vi "file_configuration.vi"(4 "force_read?":bool, 6 "custom_file":path, 7 "command":T1=enum."read_config", 8 "error in (no error)":errorcluster, 10 "project_file":path, 11 "config in":T2) -> (0 "error out":errorcluster, 3 "config out":T2)   [LabVIEW 2015, in "lv-builder-default.lvlib"]
doc: "This VI is able to read/write configuration from all the associated modules defined in the master data cluster. It also acts as a functional global/data store in the event that no data has changed since the last write. It will self-initialize and well set an internal flag in the event an error is encountered when reading. If no command is provided, it will default to the read command."
uses:
  lv-builder-default.lvlib
  _controls/configuration.ctl
  _controls/command_configuration.ctl
  lv-build/lv-build.lvlib
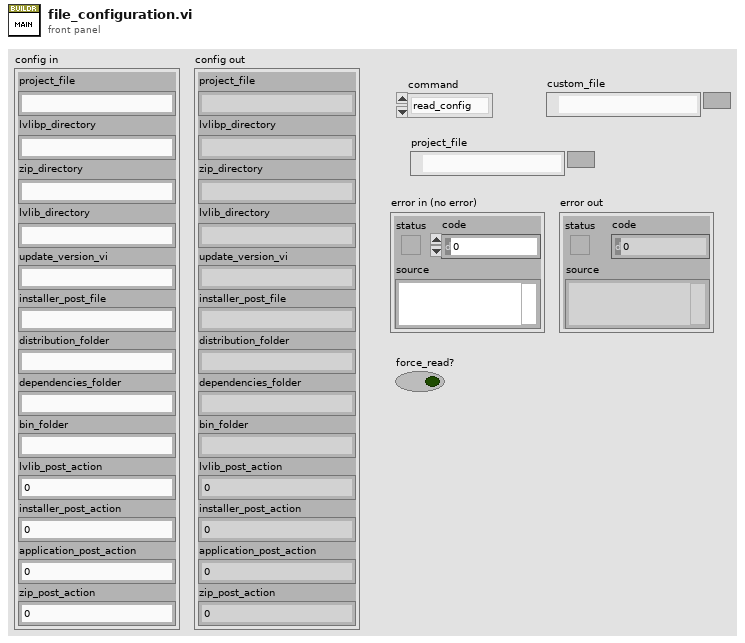
[diagram p1: front panel]
types:
  T1 = typedef "lv-builder-default.lvlib/command_configuration.ctl" = enum16{"<config_command>", "read_config", "write_config", "<null>"}
  T2 = typedef "lv-builder-default.lvlib/configuration.ctl" = cluster{"project_file":string, "lvlibp_directory":string, "zip_directory":string, "lvlib_directory":string, "update_version_vi":string, "installer_post_file":string, "distribution_folder":string, "dependencies_folder":string, "bin_folder":string, "lvlib_post_action":u16, "installer_post_action":u16, "application_post_action":u16, "zip_post_action":u16}
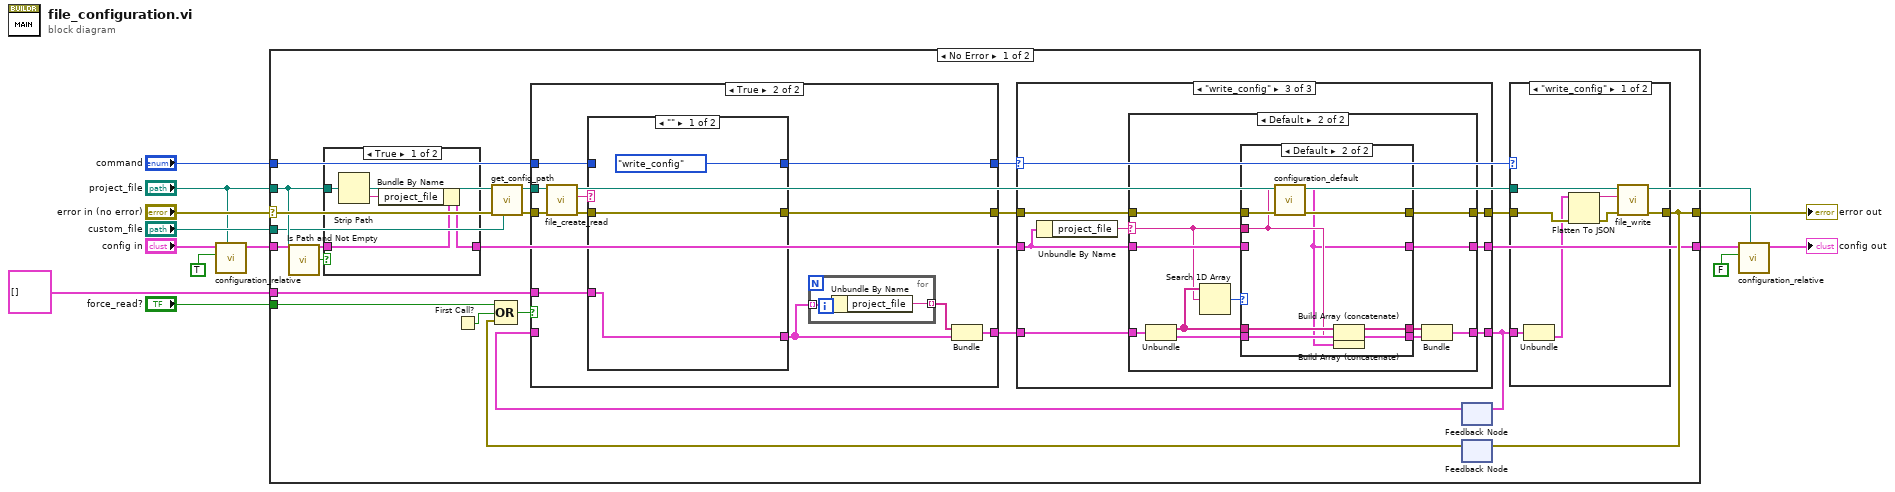
[diagram p0: block diagram]
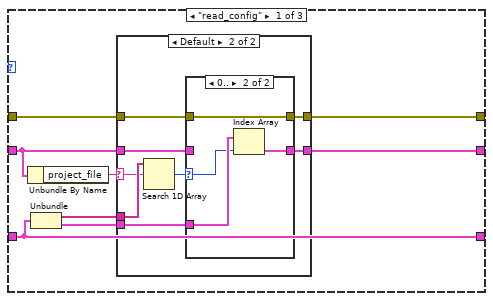
[diagram p3: hidden frame]
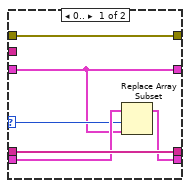
[diagram p8: hidden frame]
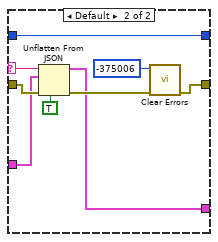
[diagram p10: hidden frame]
diagram:
  n1 = call "configuration_relative.vi"("project_file"="project_file", "to_relative"=TRUE, "configuration in"="config in") -> ("configuration out"=w3:T2)  [unwired: 8 in]
  n2 = case shown="No Error" "error in (no error)" {
    selector: "error in (no error)" -> [w19 w139]
    tunnel: "command" -> [w28 _]
    tunnel: [w35 w139] -> w10
    tunnel: w3 -> [w21 _]
    tunnel: "custom_file" -> [w14 _]
    tunnel: [w26 _] -> w6
    tunnel: "force_read?" -> [w32 _]
    tunnel: T2[] [] ("default") -> [w29 _]
    tunnel: "project_file" -> [w15 _]
    frame No Error {
      n3 = call <vilib>:"Is Path and Not Empty.vi"("path"=w15) -> ("Is Path and Not Empty?"=w16:bool)  [unwired: 4 in]
      n4 = case shown="True" w16 {
        tunnel: w21 -> [w39 w40]
        tunnel: [w38 w40] -> w17
        tunnel: w15 -> [w37 _]
        frame True {
          n5 = Strip Path(path=w37) -> (name=w36:string)  [unwired: 1 out]
          n6 = Bundle By Name(cluster=w39, "project_file"=w36) -> (w38:T2)
        }
        frame False {
        }
      }
      n7 = First Call?() -> (First Call?: T/F=w33:bool)
      n8 = call "get_config_path.vi"("custom_path"=w14, "error in (no error)"=w19, "project_file"=w15) -> ("error out"=w18:errorcluster, "lv_build_config_path"=w20:path)  [unwired: 7 in]
      n9 = feedback #1() -> (w30:cluster{string[], "default":T2[]})  [unwired: 1 in]
      n10 = feedback #2() -> (w34:errorcluster)  [unwired: 1 in]
      n11 = Compound Arithmetic op=OR(w32, w33, w34) -> (w31:bool)
      n12 = case shown="True" w31 {
        tunnel: w30 -> [w105 _]
        tunnel: w18 -> [w104 w114]
        tunnel: w20 -> [_ w115]
        tunnel: [w104 w112] -> w24
        tunnel: w29 -> [_ w116]
        tunnel: w28 -> [w103 w111]
        tunnel: [w103 w110] -> w25
        tunnel: [w105 w108] -> w27
        frame False {
        }
        frame True {
          n13 = call "file_create_read.vi"("error in (no error)"=w114, "config_path"=w115) -> ("error out"=w113:errorcluster, "string"=w109:string)  [unwired: 8 in]
          n14 = case shown="\"\"" w109 {
            selector: w109 -> [_ w126]
            tunnel: w116 -> [w120 w128]
            tunnel: [w120 w127] -> w107
            tunnel: w113 -> [w121 w130]
            tunnel: [w121 w122] -> w112
            tunnel: w111 -> [_ w125]
            tunnel: [command_configuration."write_config" ("command") w125] -> w110
            frame "" {
            }
            frame Default {
              n15 = Unflatten From JSON(JSON string=w126, type and defaults=w128, default null elements? (F)=TRUE, error in (no error)=w130) -> (value=w127:T2[], error out=w129:errorcluster)  [unwired: 3 in]
              n16 = call <vilib>:"Clear Errors.vi"("error in (no error)"=w129, "specific error code to clear (0: all)"=-375006) -> ("error out"=w122:errorcluster)  [unwired: 4 in, 1 out]
            }
          }
          n17 = for {
            tunnel: w107 -> [w118] mode=indexing
            tunnel: [w117] -> w106 mode=indexing
            n18 = Unbundle By Name(w118) -> ("project_file"=w117:string)
          }
          n19 = Bundle(w106, "default"=w107) -> (w108:cluster{string[], "default":T2[]})  [unwired: 1 in]
        }
      }
      n20 = case shown="\"write_config\"" w25 {
        tunnel: w17 -> [w41 w66 w70]
        tunnel: [w48 w65 w73] -> w22
        tunnel: w27 -> [w48 w65 w71]
        tunnel: [w44 w66 w67] -> w26
        tunnel: w24 -> [w43 w64 w69]
        tunnel: [w42 w64 w68] -> w23
        frame "read_config" {
          n21 = Unbundle By Name(w41) -> ("project_file"=w45:string)
          n22 = Unbundle(w48) -> (w47:string[], "default"=w46:T2[])
          n23 = case shown="Default" w45 {
            selector: w45 -> [_ w54]
            tunnel: w47 -> [_ w57]
            tunnel: w46 -> [_ w56]
            tunnel: [_ w53] -> w44
            tunnel: w43 -> [w49 w52]
            tunnel: [w49 w51] -> w42
            tunnel: w41 -> [_ w50]
            frame "" {
            }
            frame Default {
              n24 = Search 1D Array(1D array=w57, element=w54) -> (index of element=w55:i32)  [unwired: 1 in]
              n25 = case shown="0.." w55 {
                selector: w55 -> [_ w62]
                tunnel: w56 -> [_ w63]
                tunnel: [w58 w61] -> w53
                tunnel: w52 -> [w59 w60]
                tunnel: [w59 w60] -> w51
                tunnel: w50 -> [w58 _]
                frame Default {
                }
                frame 0.. {
                  n26 = Index Array(array=w63, index=w62) -> (element=w61:T2)
                }
              }
            }
          }
        }
        frame Default {
        }
        frame "write_config" {
          n27 = Unbundle By Name(w70) -> ("project_file"=w72:string)
          n28 = case shown="Default" w72 {
            selector: w72 -> [_ w80]
            tunnel: [w76 w86] -> w73
            tunnel: w70 -> [w74 w84]
            tunnel: w71 -> [w76 w82]
            tunnel: w69 -> [w75 w79]
            tunnel: [w75 w78] -> w68
            tunnel: [w74 w77] -> w67
            frame "" {
            }
            frame Default {
              n29 = Unbundle(w82) -> (w81:string[], "default"=w83:T2[])
              n30 = Search 1D Array(1D array=w81, element=w80) -> (index of element=w88:i32)  [unwired: 1 in]
              n31 = case shown="Default" w88 {
                selector: w88 -> [w91 _]
                tunnel: w83 -> [w93 w101]
                tunnel: [w92 w100] -> w87
                tunnel: w81 -> [w94 w98]
                tunnel: [w94 w99] -> w85
                tunnel: w84 -> [w89 _]
                tunnel: w80 -> [_ w96]
                tunnel: w79 -> [w90 w97]
                tunnel: [w90 w102] -> w78
                tunnel: [w89 w95] -> w77
                frame 0.. {
                  n32 = Replace Array Subset(array=w93, new element=w89, index=w91) -> (w92:T2[])
                }
                frame Default {
                  n33 = call "configuration_default.vi"("error in (no error)"=w97, "project_file"=w96) -> ("error out"=w102:errorcluster, "configuration"=w95:T2)  [unwired: 8 in]
                  n34 = Build Array (concatenate)(w98, w96) -> (w99:string[])
                  n35 = Build Array (concatenate)(w101, w95) -> (w100:T2[])
                }
              }
              n36 = Bundle(w85, "default"=w87) -> (w86:cluster{string[], "default":T2[]})  [unwired: 1 in]
            }
          }
        }
      }
      n37 = feedback-in #1(w22) -> ()
      n38 = case shown="\"write_config\"" w25 {
        tunnel: w22 -> [w134 _]
        tunnel: w23 -> [w135 w138]
        tunnel: [w132 w138] -> w35
        tunnel: w20 -> [w133 _]
        frame "write_config" {
          n39 = Unbundle(w134) -> ("default"=w131:T2[])  [unwired: 1 out]
          n40 = Flatten To JSON(anything=w131, error in (no error)=w135) -> (JSON string=w137:string, 11:w136:errorcluster)  [unwired: 1 in]
          n41 = call "file_write.vi"("error in (no error)"=w136, "string"=w137, "config_path"=w133) -> ("error out"=w132:errorcluster)  [unwired: 8 in]
        }
        frame Default {
        }
      }
      n42 = feedback-in #2(w35) -> ()
    }
    frame Error {
      # "If an error is wired in, be sure to skip over functionality to preserve the original error"
    }
  }
  "error out" <- w10
  n43 = call "configuration_relative.vi"("project_file"="project_file", "to_relative"=FALSE, "configuration in"=w6) -> ("configuration out"=→"config out":T2)  [unwired: 8 in]
